vi "segmentation.vi"(0 "unmixed ch2":dbl[][](array[numeric])=array223x128[28544 elements], 5 "segmentation method":T3={"normalize for thresholding"=TRUE, "use threshold formula"=FALSE, "threshold"=0.27000000000000013, "manual thresholding"=TRUE, "Method (clustering)"=2, "upper limit"=9000} {"Method (clustering)" items=["clustering", "entropy", "metric", "moments", "inter-class variance"]; "threshold" format="%_3g"}, 7 "image lpf":cluster{"cutoff ":dbl, "lpf":bool, "order":i32}={"cutoff "=0.20000010000000001, "lpf"=FALSE, "order"=2} {"cutoff" min=1e-07 max=0.4999 step=0.01 format="%_2g"}, 9 "post processing":T2={"truncation for ch2 masking"=[0, 0, 0, 0], "Number of Erosion"=3, "Operation"=enum."Close", "post processing"=TRUE, "move x/y"=[0, 0], "convex"=FALSE, "Connectivity 4/8 (8)"=TRUE, "Number of iterations (1)"=1, "Number of Erosion 2"=3}, 11 "input cluster":T1 {"Method (Niblack)" items=["Niblack", "Background Correction", "Sauvola"]}, 12 "Threshold Limits":cluster{"Lower value":sgl, "Upper value":sgl}={"Lower value"=-32768.0, "Upper value"=65535.0} {"Upper value" format="%.2f"; "Lower value" format="%.2f"}) -> (3 "Array":u8[][](array[numeric]), 6 "output variable":dbl=0.27000000000000013, 15 "error out":errorcluster)   [LabVIEW 2018]
uses:
  <vilib>/vision/NI_Vision_Development_Module.lvlib
panel:
  out "threshold":dbl format="%_6g"
  out "In Range?":bool
  out "error out 2":errorcluster
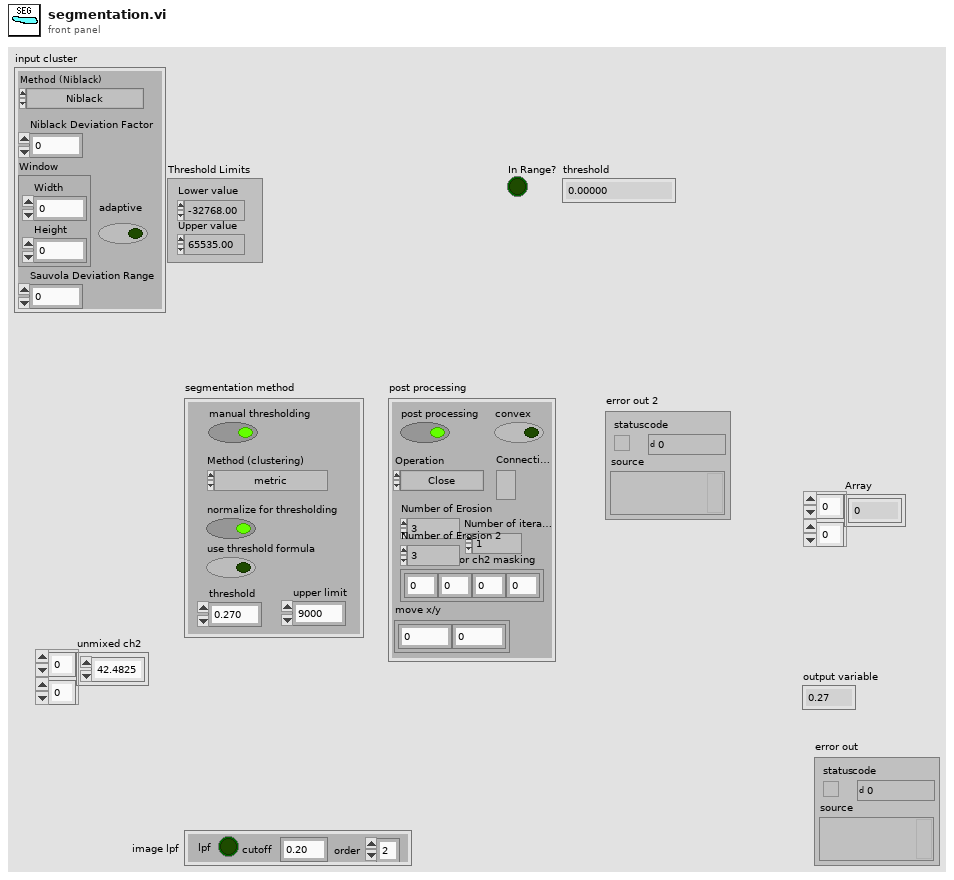
[diagram p1: front panel]
types:
  T1 = cluster{"Niblack Deviation Factor":dbl, "Window":cluster{"Width":i32, "Height":i32}, "Sauvola Deviation Range":dbl, "adaptive":bool, "Method (Niblack)":u32}
  T2 = cluster{"truncation for ch2 masking":i32[], "Number of Erosion":i32, "Operation":enum32{"AutoM", "Close", "Dilate", "Erode", "Gradient", "Gradient out", "Gradient in", "Hit miss", "Open", "PClose", "POpen", "Thick", "Thin"}, "post processing":bool, "move x/y":i32[], "convex":bool, "Connectivity 4/8 (8)":bool, "Number of iterations (1)":i32, "Number of Erosion 2":i32}
  T3 = cluster{"normalize for thresholding":bool, "use threshold formula":bool, "threshold":dbl, "manual thresholding":bool, "Method (clustering)":i32, "upper limit":i32}
  T4 = typedef "Image Type" = u32
  T5 = typedef "IMAQ Image.ctl" = refnum<image>
  T6 = enum32{"AutoM", "Close", "Dilate", "Erode", "Gradient", "Gradient out", "Gradient in", "Hit miss", "Open", "PClose", "POpen", "Thick", "Thin"}
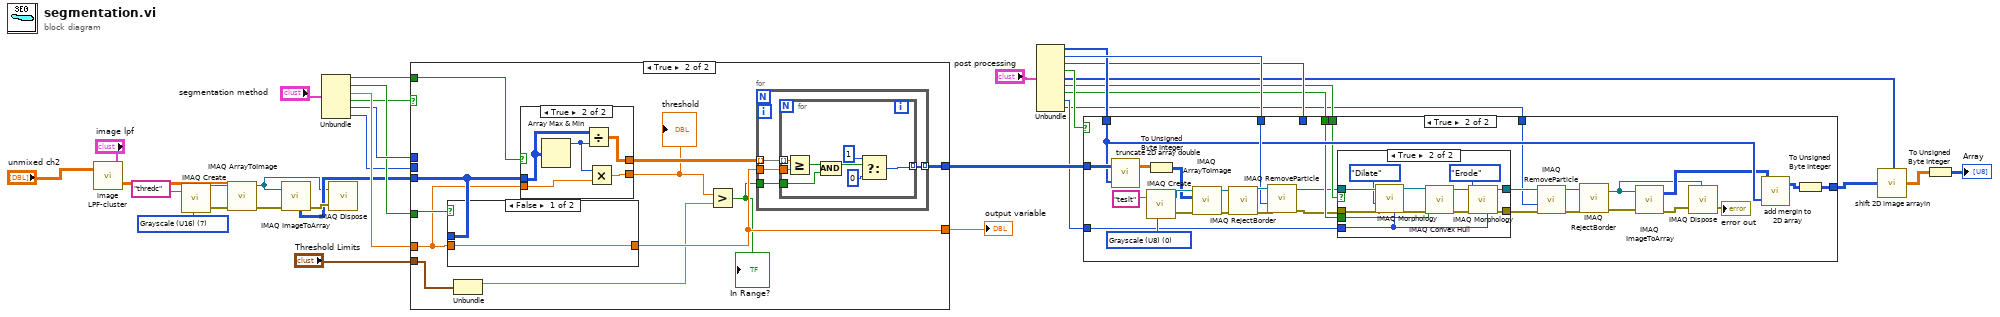
[diagram p0: block diagram]
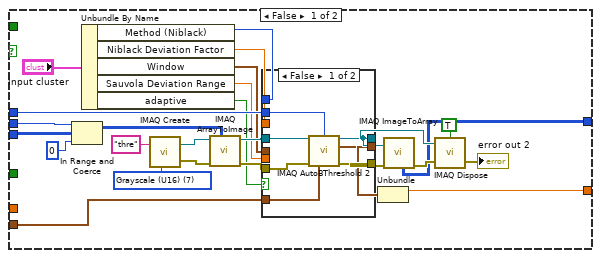
[diagram p2: hidden frame]
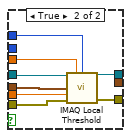
[diagram p3: hidden frame]
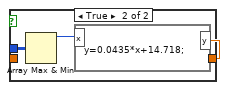
[diagram p4: hidden frame]
diagram:
  w14 = T4 7 items=["Grayscale (U8)", "Grayscale (I16)", "Grayscale (SGL)", "Complex (CSG)", "RGB (U32)", "HSL (U32)", "RGB (U64)", "Grayscale (U16)"] ("Image Type")
  n1 = call "image LPF-cluster.vi"("image lpf"="image lpf", "input"="unmixed ch2") -> ("output"=w11:dbl[][])  [unwired: 1 in]
  n2 = call "IMAQ Create"("Image Name"="thredc", "Image Type"=w14) -> ("New Image"=w15:T5, "error out"=w13:errorcluster)  [unwired: 3 in]
  n3 = call "IMAQ ArrayToImage"("Image Pixels (U16)"=w11, "error in (no error)"=w13, "Image"=w15) -> ("error out"=w8:errorcluster, "Image Out"=w9:T5)  [unwired: 7 in]
  n4 = call "IMAQ ImageToArray"("error in (no error)"=w8, "Image"=w9) -> ("Image Pixels (U16)"=w10:u16[][], "error out"=w12:errorcluster)  [unwired: 2 in, 3 out]
  n5 = Unbundle("segmentation method") -> ("normalize for thresholding"=w28:bool, "use threshold formula"=w20:bool, "threshold"=w27:dbl, "manual thresholding"=w19:bool, "Method (clustering)"=w26:i32, "upper limit"=w17:i32)
  n6 = call "IMAQ Dispose"("Image"=w9, "error in (no error)"=w12) -> ()  [unwired: 4 in, 1 out]
  n7 = case shown="True" w19 {
    tunnel: w10 -> [w44 w85]
    tunnel: [w48 w84] -> w30
    tunnel: w28 -> [_ w83]
    tunnel: w20 -> [_ w82]
    tunnel: w26 -> [w52 _]
    tunnel: w27 -> [_ w77]
    tunnel: [w46 w80] -> w18
    tunnel: w17 -> [w42 _]
    tunnel: "Threshold Limits" -> [w35 w81]
    frame False {
      w58 = T4 7 items=["Grayscale (U8)", "Grayscale (I16)", "Grayscale (SGL)", "Complex (CSG)", "RGB (U32)", "HSL (U32)", "RGB (U64)", "Grayscale (U16)"] ("Image Type")
      n8 = In Range and Coerce(upper limit=w42, x=w44, lower limit=0) -> (coerced(x)=w43:i32[][])  [unwired: 1 out]
      n9 = Unbundle By Name("input cluster") -> ("Method (Niblack)"=w36:u32, "Niblack Deviation Factor"=w38:dbl, "Window"=w40:cluster{"Width":i32, "Height":i32}, "Sauvola Deviation Range"=w39:dbl, "adaptive"=w37:bool)
      n10 = call "IMAQ Create"("Image Name"="thre", "Image Type"=w58) -> ("New Image"=w57:T5, "error out"=w59:errorcluster)  [unwired: 3 in]
      n11 = call "IMAQ ArrayToImage"("Image Pixels (U16)"=w43, "error in (no error)"=w59, "Image"=w57) -> ("error out"=w54:errorcluster, "Image Out"=w55:T5)  [unwired: 7 in]
      n12 = case shown="False" w37 {
        tunnel: w55 -> [w67 w74]
        tunnel: w54 -> [w66 w72]
        tunnel: [w65 w71] -> w53
        tunnel: w52 -> [w64 _]
        tunnel: [w63 w73] -> w49
        tunnel: [w62 _] -> w47
        tunnel: w36 -> [_ w75]
        tunnel: w40 -> [_ w70]
        tunnel: w39 -> [_ w69]
        tunnel: w38 -> [_ w68]
        tunnel: w35 -> [w61 _]
        frame False {
          n13 = call "IMAQ AutoBThreshold 2"("Image Src"=w67, "Method (clustering)"=w64, "error in (no error)"=w66, "Threshold Limits"=w61) -> ("Image Dst Out"=w63:T5, "Threshold Range Out"=w62:cluster{"Lower value":sgl, "Upper value":sgl}, "error out"=w65:errorcluster)  [unwired: 9 in]
        }
        frame True {
          n14 = call "IMAQ Local Threshold"("Image Src"=w74, "Method (Niblack)"=w75, "Window Size (32x32)"=w70, "Sauvola Deviation Range"=w69, "error in (no error)"=w72, "Niblack/Sauvola Deviation Factor (0.2)"=w68) -> ("Image Dst Out"=w73:T5, "error out"=w71:errorcluster)  [unwired: 8 in]
        }
      }
      n15 = Unbundle(w47) -> ("Lower value"=w46:sgl)  [unwired: 1 out]
      n16 = call "IMAQ ImageToArray"("error in (no error)"=w53, "Image"=w49) -> ("Image Pixels (U16)"=w48:u16[][], "error out"=w60:errorcluster)  [unwired: 2 in, 3 out]
      n17 = call "IMAQ Dispose"("All Images? (No)"=TRUE, "Image"=w49, "error in (no error)"=w60) -> ("error out"=→"error out 2":errorcluster)  [unwired: 3 in]
    }
    frame True {
      n18 = case shown="False" w82 {
        tunnel: w85 -> [_ w89]
        tunnel: [w87 w88] -> w80
        tunnel: w77 -> [w87 _]
        frame False {
        }
        frame True {
          n19 = Array Max & Min(array=w89) -> (max value=w90:u16)  [unwired: 3 out]
          n20 = formula code="y=0.0435*x+14.718;"("x"=w90) -> ("y"=w88:dbl)
        }
      }
      n21 = Unbundle(w81) -> ("Lower value"=w79:sgl)  [unwired: 1 out]
      n22 = case shown="True" w83 {
        tunnel: [w92 w97] -> w86
        tunnel: w85 -> [w92 w96]
        tunnel: w77 -> [w91 w94]
        tunnel: [w91 w93] -> w76
        frame False {
        }
        frame True {
          n23 = Array Max & Min(array=w96) -> (max value=w95:u16)  [unwired: 3 out]
          n24 = Divide(x=w96, y=w95) -> (x/y=w97:dbl[][])
          n25 = Multiply(x=w95, y=w94) -> (x*y=w93:dbl)
        }
      }
      "threshold" <- w76
      n26 = Greater?(x=w76, y=w79) -> (0:w78:bool)
      "In Range?" <- w78
      n27 = for {
        tunnel: w86 -> [w101] mode=indexing
        tunnel: [w99] -> w84 mode=indexing
        tunnel: w80 -> [w100]
        tunnel: w78 -> [w98]
        n28 = for {
          tunnel: w101 -> [w109] mode=indexing
          tunnel: [w105] -> w99 mode=indexing
          tunnel: w100 -> [w104]
          tunnel: w98 -> [w102]
          n29 = Greater Or Equal?(x=w109, y=w104) -> (x >= y?=w108:bool)
          n30 = And(x=w108, y=w102) -> (x .and. y?=w103:bool)
          n31 = Select(t=u8 1, s=w103, f=u8 0) -> (s? t:f=w105:u8)
        }
      }
    }
  }
  "output variable" <- w18
  n32 = Unbundle("post processing") -> ("truncation for ch2 masking"=w22:i32[], "Number of Erosion"=w23:i32, "Operation"=w21:T6, "post processing"=w24:bool, "move x/y"=w3:i32[], "convex"=w7:bool, "Connectivity 4/8 (8)"=w6:bool, "Number of iterations (1)"=w5:i32, "Number of Erosion 2"=w4:i32)
  n33 = case shown="True" w24 {
    tunnel: w30 -> [w110 w127]
    tunnel: [w110 w134] -> w2
    tunnel: w23 -> [_ w126]
    tunnel: w21 -> [_ _]
    tunnel: w22 -> [_ w125]
    tunnel: w7 -> [_ w123]
    tunnel: w6 -> [_ w122]
    tunnel: w5 -> [_ w112]
    tunnel: w4 -> [_ w119]
    frame False {
    }
    frame True {
      w138 = T4 0 items=["Grayscale (U8)", "Grayscale (I16)", "Grayscale (SGL)", "Complex (CSG)", "RGB (U32)", "HSL (U32)", "RGB (U64)", "Grayscale (U16)"] ("Image Type")
      n34 = call "truncate 2D array double.vi"("b-t-l-r"=w125, "Array in"=w127) -> ("Array out"=w137:dbl[][])  [unwired: 1 in]
      n35 = To Unsigned Byte Integer(number=w137) -> (unsigned 8bit integer=w132:u8[][])
      n36 = call "IMAQ Create"("Image Name"="teslt", "Image Type"=w138) -> ("New Image"=w139:T5, "error out"=w133:errorcluster)  [unwired: 3 in]
      n37 = call "IMAQ ArrayToImage"("error in (no error)"=w133, "Image Pixels (U8)"=w132, "Image"=w139) -> ("error out"=w129:errorcluster, "Image Out"=w130:T5)  [unwired: 7 in]
      n38 = call "IMAQ RejectBorder"("error in (no error)"=w129, "Image Src"=w130) -> ("error out"=w131:errorcluster, "Image Dst Out"=w136:T5)  [unwired: 4 in]
      n39 = call "IMAQ RemoveParticle"("error in (no error)"=w131, "Number of Erosion"=w126, "Image Src"=w136) -> ("error out"=w111:errorcluster, "Image Dst Out"=w113:T5)  [unwired: 7 in]
      n40 = case shown="True" w123 {
        tunnel: w111 -> [w141 w147]
        tunnel: w113 -> [w142 w151]
        tunnel: [w141 w145] -> w121
        tunnel: [w142 w148] -> w120
        tunnel: w122 -> [_ w153]
        tunnel: w112 -> [_ w152]
        frame False {
        }
        frame True {
          n41 = call "IMAQ Morphology"("Number of iterations (1)"=w152, "error in (no error)"=w147, "Operation"=T6."Dilate", "Image Src"=w151) -> ("Image Dst Out"=w150:T5)  [unwired: 6 in, 1 out]
          n42 = call "IMAQ Convex Hull"("error in (no error)"=w147, "Connectivity 4/8 (8)"=w153, "Image Src"=w150) -> ("error out"=w146:errorcluster, "Image Dst Out"=w149:T5)  [unwired: 7 in]
          n43 = call "IMAQ Morphology"("Number of iterations (1)"=w152, "error in (no error)"=w146, "Operation"=T6."Erode", "Image Src"=w149) -> ("error out"=w145:errorcluster, "Image Dst Out"=w148:T5)  [unwired: 6 in]
        }
      }
      n44 = call "IMAQ RemoveParticle"("error in (no error)"=w121, "Number of Erosion"=w119, "Image Src"=w120) -> ("error out"=w117:errorcluster, "Image Dst Out"=w116:T5)  [unwired: 7 in]
      n45 = call "IMAQ RejectBorder"("error in (no error)"=w117, "Image Src"=w116) -> ("error out"=w115:errorcluster, "Image Dst Out"=w114:T5)  [unwired: 4 in]
      n46 = call "IMAQ ImageToArray"("error in (no error)"=w115, "Image"=w114) -> ("error out"=w118:errorcluster, "Image Pixels (U8)"=w124:u8[][])  [unwired: 2 in, 3 out]
      n47 = call "IMAQ Dispose"("Image"=w114, "error in (no error)"=w118) -> ("error out"=→"error out":errorcluster)  [unwired: 4 in]
      n48 = call "add mergin to 2D array.vi"("mergin array"=w125, "Array in"=w124) -> ("Array out"=w135:u8[][])  [unwired: 1 in]
      n49 = To Unsigned Byte Integer(number=w135) -> (unsigned 8bit integer=w134:u8[][])
    }
  }
  n50 = call "shift 2D image arrayin.vi"("Array in"=w2, "shift"=w3) -> ("Array out"=w32:dbl[][])
  n51 = To Unsigned Byte Integer(number=w32) -> (unsigned 8bit integer=→"Array":u8[][])
